vi "Update_Vision_Tuning.vi"(10 "New Filter":T1, 11 "LV to OpenCV":dbl) -> ()   [LabVIEW 2020]
uses:
  <vilib>/Rock Robotics/Network Tables/NT Write Number.vi
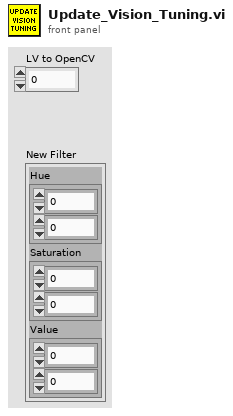
[diagram p1: front panel]
types:
  T1 = cluster{"Hue":cluster{dbl, dbl}, "Saturation":cluster{dbl, dbl}, "Value":cluster{dbl, dbl}}
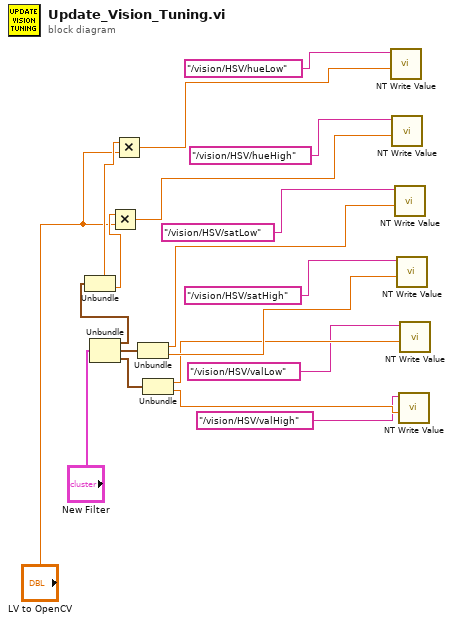
[diagram p0: block diagram]
diagram:
  n1 = Unbundle("New Filter") -> ("Hue"=w9:cluster{dbl, dbl}, "Saturation"=w14:cluster{dbl, dbl}, "Value"=w15:cluster{dbl, dbl})
  n2 = Unbundle(w9) -> (w10:dbl, w11:dbl)
  n3 = Multiply(x=w11, y="LV to OpenCV") -> (x*y=w13:dbl)
  n4 = Multiply(x=w10, y="LV to OpenCV") -> (x*y=w12:dbl)
  n5 = Unbundle(w14) -> (w18:dbl, w19:dbl)
  n6 = Unbundle(w15) -> (w16:dbl, w17:dbl)
  n7 = call-poly <vilib>:"NT Write Value.vi"("value"=w12, "name"="/vision/HSV/hueLow") -> ()  [unwired: 9 in, 1 out]
  n8 = call-poly <vilib>:"NT Write Value.vi"("value"=w13, "name"="/vision/HSV/hueHigh") -> ()  [unwired: 9 in, 1 out]
  n9 = call-poly <vilib>:"NT Write Value.vi"("value"=w18, "name"="/vision/HSV/satLow") -> ()  [unwired: 9 in, 1 out]
  n10 = call-poly <vilib>:"NT Write Value.vi"("value"=w19, "name"="/vision/HSV/satHigh") -> ()  [unwired: 9 in, 1 out]
  n11 = call-poly <vilib>:"NT Write Value.vi"("value"=w17, "name"="/vision/HSV/valHigh") -> ()  [unwired: 9 in, 1 out]
  n12 = call-poly <vilib>:"NT Write Value.vi"("value"=w16, "name"="/vision/HSV/valLow") -> ()  [unwired: 9 in, 1 out]
